vi "Hard_AWG_5421_Standard_Function.vi"(8 "error in (no error)":errorcluster caption="entrée d'erreur (pas d'erreur)") -> (0 "error out":errorcluster caption="sortie d'erreur")   [LabVIEW 2020]
doc: "This example shows the Standard Function output mode. \n\nIt also shows some of the parameters which can be changed on the fly."
uses:
  <instrlib>/niFgen/niFgen.llb/niFgen Output Mode.ctl
panel:
  in  "Gain":dbl=0.31 caption="Gain (0 to 1)" min=0.0 max=1.0
  in  "stop":bool
  in  "Waveform":u32(slide)
  in  "Update":bool
  in  "DC Offset (V)":dbl
  in  "Amplitude (Vp-p)":dbl=0.04 min=0.01 max=10.0
  in  "frequency (Hz)":dbl=2000000.0 caption="Frequency (Hz)" format="%#_6p"
  in  "Resource Name":refnum<k15>="AWG_5421"
  in  "Start Phase":dbl format="%.2f"
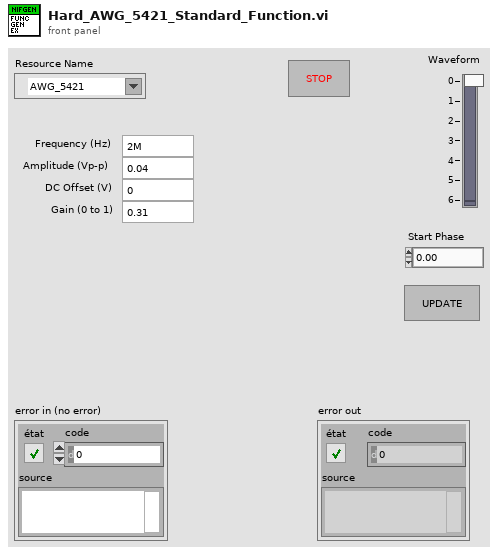
[diagram p1: front panel]
types:
  T1 = typedef "niFgen Output Mode.ctl" = u32
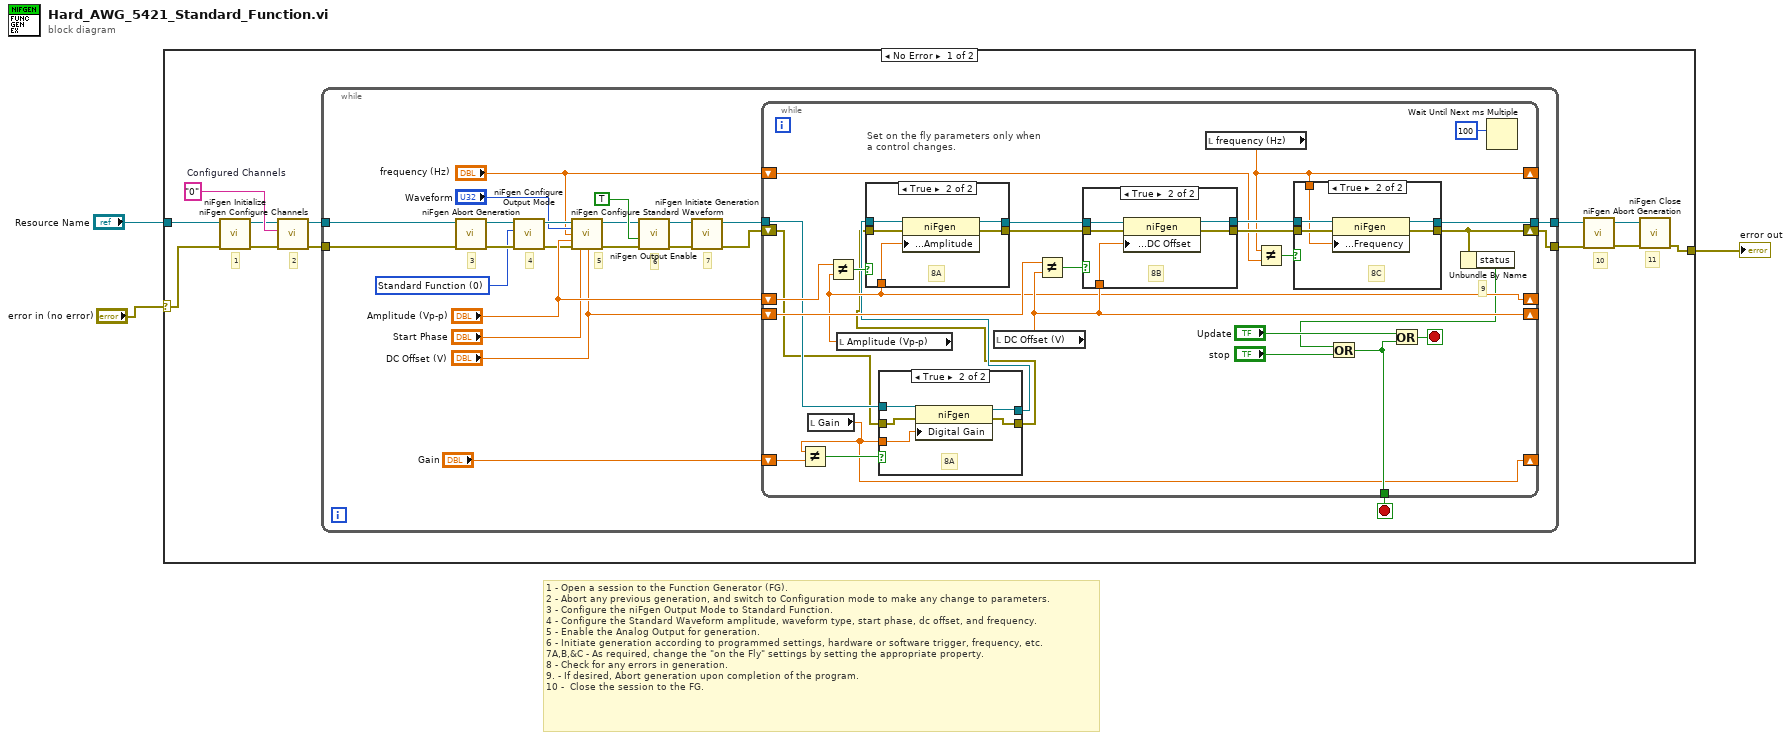
[diagram p0: block diagram]
diagram:
  # "1 - Open a session to the Function Generator (FG).\n2 - Abort any previous generation, and switch to Configuration mode to make any change to parameters.\n3 - Configure the niFgen Output Mode to Standard Function.\n4 - Configure the Standard Waveform amplitude, waveform type, start phase, dc offset, and frequency.\n5 - Enable the Analog Output for generation.\n6 - Initiate generation according to programmed settings, hardware or software trigger, frequency, etc.\n7A,B,&C - As required, change the \"on the Fly\" settings by setting the appropriate property.\n8 - Check for any errors in generation.\n9. - If desired, Abort generation upon completion of the program.\n10 -  Close the session to the FG."
  n1 = case shown="No Error" "error in (no error)" {
    selector: "error in (no error)" -> [w5 w95]
    tunnel: "Resource Name" -> [w11 _]
    tunnel: [w4 w95] -> w1
    frame No Error {
      w10 = "0"  # Configured Channels
      # "2"
      # "10"
      # "11"
      # "1"
      n2 = call <instrlib>:"niFgen Initialize.vi"("error in (no error)"=w5, "Resource Name"=w11) -> ("error out"=w9:errorcluster, "Instrument Handle Out"=w6:refnum<k15>)  [unwired: 8 in]
      n3 = call <instrlib>:"niFgen Configure Channels.vi"("error in (no error)"=w9, "Channels"=w10, "Instrument Handle"=w6) -> ("error out"=w8:errorcluster, "Instrument Handle Out"=w7:refnum<k15>)  [unwired: 7 in]
      n4 = while {
        tunnel: w8 -> [w21]
        tunnel: w7 -> [w22]
        tunnel: [w37] -> w14
        tunnel: [w38] -> w15
        stop <- w36 stop-if-true
        w20 = T1 0 items=["Standard Function", "Frequency List", "Arbitrary Waveform", "Arbitrary Sequence", "Script"] ("output mode")
        # "7"
        # "6"
        # "5"
        # "4"
        # "3"
        n5 = call <instrlib>:"niFgen Abort Generation.vi"("error in (no error)"=w21, "Instrument Handle"=w22) -> ("error out"=w29:errorcluster, "Instrument Handle Out"=w28:refnum<k15>)  [unwired: 8 in]
        n6 = call <instrlib>:"niFgen Configure Output Mode.vi"("error in (no error)"=w29, "Output Mode (default: 0=Standard Function)"=w20, "Instrument Handle"=w28) -> ("error out"=w33:errorcluster, "Instrument Handle Out"=w31:refnum<k15>)  [unwired: 6 in]
        n7 = call <instrlib>:"niFgen Configure Standard Waveform.vi"("Instrument Handle"=w31, "Waveform"="Waveform", "Frequency"="frequency (Hz)", "Amplitude"="Amplitude (Vp-p)", "error in (no error)"=w33, "Start Phase"="Start Phase", "DC Offset"="DC Offset (V)") -> ("Instrument Handle Out"=w18:refnum<k15>, "error out"=w19:errorcluster)  [unwired: 7 in]
        n8 = call <instrlib>:"niFgen Output Enable.vi"("error in (no error)"=w19, "Output Enable (default: True)"=TRUE ("output enable"), "Instrument Handle"=w18) -> ("error out"=w32:errorcluster, "Instrument Handle Out"=w30:refnum<k15>)  [unwired: 7 in]
        n9 = call <instrlib>:"niFgen Initiate Generation.vi"("error in (no error)"=w32, "Instrument Handle"=w30) -> ("error out"=w25:errorcluster, "Instrument Handle Out"=w26:refnum<k15>)  [unwired: 8 in]
        n10 = while {
          tunnel: [w50] -> w36
          shift-left: w25 -> [w41]
          shift-right: [w49] -> w37
          shift-left: "DC Offset (V)" -> [w60]
          shift-right: [w55] -> _
          shift-left: "Amplitude (Vp-p)" -> [w61]
          shift-right: [w53] -> _
          shift-left: "frequency (Hz)" -> [w57]
          shift-right: [w46] -> _
          tunnel: [w52] -> w38
          tunnel: w26 -> [w43]
          shift-right: [w39] -> _
          shift-left: "Gain" -> [w45]
          stop <- w65 stop-if-true
          # "9"
          # "Set on the fly parameters only when \na control changes."
          n11 = local read "Gain"() -> (w39:dbl)
          n12 = Not Equal?(x=w39, y=w45) -> (x != y?=w44:bool)
          n13 = local read "Amplitude (Vp-p)"() -> (w53:dbl)
          n14 = Not Equal?(x=w61, y=w53) -> (x != y?=w47:bool)
          n15 = case shown="True" w44 {
            tunnel: [w68 w73] -> w42
            tunnel: [w67 w72] -> w40
            tunnel: w39 -> [_ w71]
            tunnel: w43 -> [w68 w70]
            tunnel: w41 -> [w67 w69]
            frame False {
            }
            frame True {
              # "8A"
              n16 = property class="niFgen"(reference=w70, error in=w69, "Digital Gain"=w71) -> (reference out=w73:refnum<k15>, error out=w72:errorcluster)
            }
          }
          n17 = case shown="True" w47 {
            tunnel: w42 -> [w89 w93]
            tunnel: [w89 w91] -> w64
            tunnel: [w88 w90] -> w62
            tunnel: w40 -> [w88 w92]
            tunnel: w53 -> [_ w94]
            frame False {
            }
            frame True {
              # "8A"
              n18 = property class="niFgen"(reference=w93, error in=w92, "Standard Function:Amplitude"=w94) -> (reference out=w91:refnum<k15>, error out=w90:errorcluster)
            }
          }
          n19 = local read "DC Offset (V)"() -> (w55:dbl)
          n20 = Not Equal?(x=w60, y=w55) -> (x != y?=w59:bool)
          n21 = case shown="True" w59 {
            tunnel: w64 -> [w82 w87]
            tunnel: [w82 w86] -> w63
            tunnel: w62 -> [w81 w83]
            tunnel: w55 -> [_ w84]
            tunnel: [w81 w85] -> w58
            frame False {
            }
            frame True {
              # "8B"
              n22 = property class="niFgen"(reference=w87, error in=w83, "Standard Function:DC Offset"=w84) -> (reference out=w86:refnum<k15>, error out=w85:errorcluster)
            }
          }
          n23 = local read "frequency (Hz)"() -> (w46:dbl)
          n24 = Not Equal?(x=w46, y=w57) -> (x != y?=w56:bool)
          n25 = case shown="True" w56 {
            tunnel: [w75 w78] -> w52
            tunnel: [w74 w77] -> w49
            tunnel: w63 -> [w75 w80]
            tunnel: w58 -> [w74 w79]
            tunnel: w46 -> [_ w76]
            frame False {
            }
            frame True {
              # "8C"
              n26 = property class="niFgen"(reference=w80, error in=w79, "Standard Function:Standard Function Mode:Frequency"=w76) -> (reference out=w78:refnum<k15>, error out=w77:errorcluster)
            }
          }
          n27 = Unbundle By Name(w49) -> ("status"=w48:bool)
          n28 = Or(x=w48, y="stop") -> (x .or. y?=w50:bool)
          n29 = Or(x="Update", y=w50) -> (x .or. y?=w65:bool)
          n30 = Wait Until Next ms Multiple(millisecond multiple=u32 100) -> ()  [unwired: 1 out]
        }
      }
      n31 = call <instrlib>:"niFgen Abort Generation.vi"("error in (no error)"=w14, "Instrument Handle"=w15) -> ("error out"=w12:errorcluster, "Instrument Handle Out"=w13:refnum<k15>)  [unwired: 8 in]
      n32 = call <instrlib>:"niFgen Close.vi"("error in (no error)"=w12, "Instrument Handle"=w13) -> ("error out"=w4:errorcluster)  [unwired: 9 in]
    }
    frame Error {
    }
  }
  "error out" <- w1
